vi "niDTS GNSS RF Test Configure.vi"(0 "Template Tx Test Handle in":T2, 7 "Parameters":T1 {"External Attenuation (dB)" format="%.1g"; "Power (dBm)" format="%.1g"}, 11 "error in (no error)":errorcluster) -> (4 "Template Tx Test Handle out":T2, 15 "error out":errorcluster)   [LabVIEW 2014, in "niDTS GNSS.lvlib"]
uses:
  niDTS GNSS.lvlib
  Includes/niDTS GNSS RF Test INC Handle.ctl
  Objects/BASE_class/niDTS GNSS RF Test.lvclass
  Includes/niDTS GNSS RF Test INC Parameters.ctl
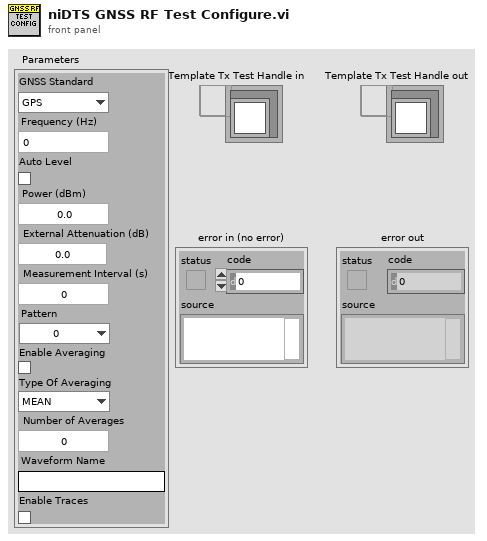
[diagram p1: front panel]
types:
  T1 = typedef "niDTS GNSS.lvlib/niDTS GNSS RF Test INC Parameters.ctl" = cluster{"GNSS Standard":enum16{"GPS", "GLONASS", "Galileo", "Beidou"}, "Frequency (Hz)":dbl, "Auto Level":bool, "Power (dBm)":dbl, "External Attenuation (dB)":dbl, "Measurement Interval (s)":dbl, "Pattern":enum16{"0", "1", "01", "00001111", "PN9"}, "Enable Averaging":bool, "Type Of Averaging":enum16{"MEAN", "MAX", "MIN", "MAXMIN"}, "Number of Averages":i32, "Waveform Name":string, "Enable Traces":bool}
  T2 = typedef "niDTS GNSS.lvlib/niDTS GNSS RF Test INC Handle.ctl" = refnum<data-value>
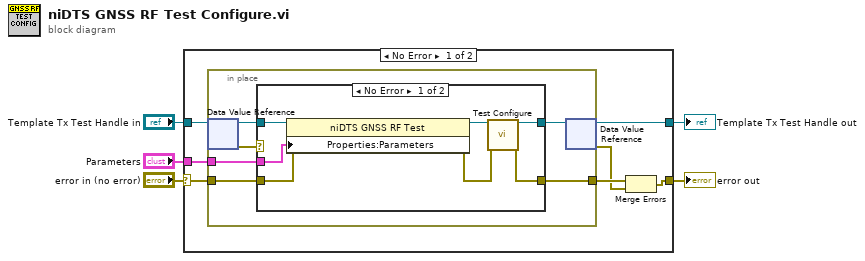
[diagram p0: block diagram]
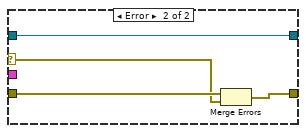
[diagram p2: hidden frame]
diagram:
  n1 = case shown="No Error" "error in (no error)" {
    selector: "error in (no error)" -> [w9 w31]
    tunnel: "Parameters" -> [w12 _]
    tunnel: "Template Tx Test Handle in" -> [w11 w30]
    tunnel: [w10 w30] -> w3
    tunnel: [w8 w31] -> w2
    frame No Error {
      n2 = in-place {
        in-place-border: w9 -> [w15]
        in-place-border: [w14] -> w7
        in-place-border: w12 -> [w13]
        n3 = in-place-dvr #1(w11) -> (w17:refnum<class "niDTS GNSS RF Test.lvclass">, w18:errorcluster)
        n4 = case shown="No Error" w18 {
          selector: w18 -> [_ w27]
          tunnel: w17 -> [w25 w29]
          tunnel: [w21 w29] -> w16
          tunnel: w15 -> [w24 w28]
          tunnel: [w22 w26] -> w14
          tunnel: w13 -> [w19 _]
          frame No Error {
            n5 = property class="niDTS GNSS RF Test"(reference=w25, error in=w24, "Properties:Parameters"=w19) -> (reference out=w20:refnum<class "niDTS GNSS RF Test.lvclass">, error out=w23:errorcluster)
            n6 = call-dynamic "Test Configure.vi"("Template RF Test in"=w20, "error in (no error)"=w23) -> ("Template RF Test out"=w21:refnum<class "niDTS GNSS RF Test.lvclass">, "error out"=w22:errorcluster)  [unwired: 12 in]
          }
          frame Error {
            n7 = Merge Errors(w28, w27) -> (w26:errorcluster)
          }
        }
        n8 = in-place-dvr #1(w16) -> (w10:T2, w6:errorcluster)
      }
      n9 = Merge Errors(w7, w6) -> (w8:errorcluster)
    }
    frame Error {
    }
  }
  "Template Tx Test Handle out" <- w3
  "error out" <- w2
